vi "Move SBlock Down.vi"(8 "error in (no error)":errorcluster, 10 "index":i32, 11 "Sequence of SBlocks in":refnum<class "Sequence of SBlocks.lvclass">) -> (0 "error out":errorcluster, 2 "New Index":i32, 3 "Sequence of SBlocks out":refnum<class "Sequence of SBlocks.lvclass">)   [LabVIEW 2020, in "Run Utilities.lvlib" / "Sequence of SBlocks.lvclass"]
uses:
  Sequence of SBlocks.lvclass
  Sequence of SBlocks.lvclass/Sequence of SBlocks.ctl
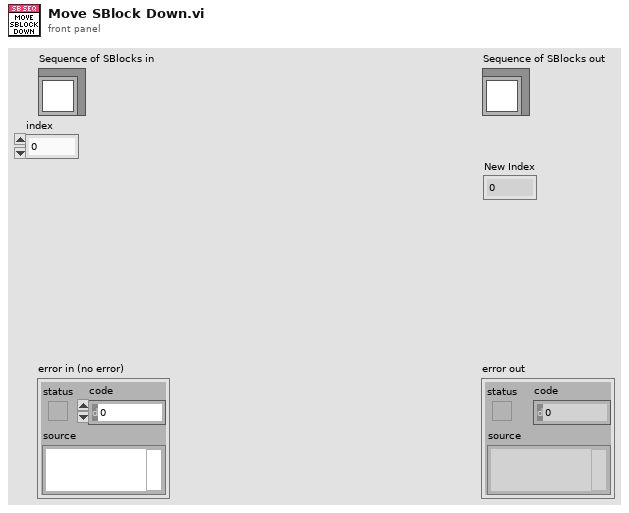
[diagram p1: front panel]
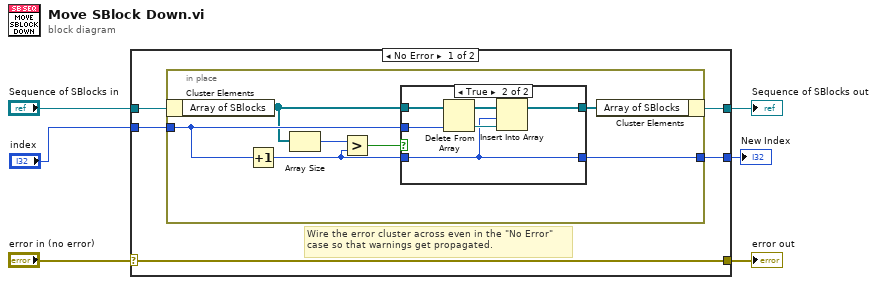
[diagram p0: block diagram]
diagram:
  n1 = case shown="No Error" "error in (no error)" {
    selector: "error in (no error)" -> [w11 w29]
    tunnel: [w11 w29] -> w5
    tunnel: [w9 w28] -> w3
    tunnel: "Sequence of SBlocks in" -> [w10 w28]
    tunnel: "index" -> [w8 w27]
    tunnel: [w7 w27] -> w1
    frame No Error {
      # "Wire the error cluster across even in the \"No Error\"\ncase so that warnings get propagated."
      n2 = in-place {
        in-place-border: w8 -> [w18]
        in-place-border: [w16] -> w7
        n3 = in-place-cluster #1(w10) -> ("Array of SBlocks"=w15:refnum<class "Schedule Block.lvclass">[])
        n4 = Increment(x=w18) -> (x+1=w13:i32)
        n5 = Array Size(array=w15) -> (size(s)=w14:i32)
        n6 = Greater?(x=w14, y=w13) -> (0:w12:bool)
        n7 = case shown="True" w12 {
          tunnel: w15 -> [w20 w26]
          tunnel: w18 -> [w19 w23]
          tunnel: [w20 w22] -> w17
          tunnel: w13 -> [_ w21]
          tunnel: [w19 w21] -> w16
          frame False {
          }
          frame True {
            n8 = Delete From Array(array=w26, index=w23) -> (deleted portion=w24:refnum<class "Schedule Block.lvclass">, array with subset deleted=w25:refnum<class "Schedule Block.lvclass">[])  [unwired: 1 in]
            n9 = Insert Into Array(array=w25, index=w21, new element=w24) -> (w22:refnum<class "Schedule Block.lvclass">[])
          }
        }
        n10 = in-place-cluster #1("Array of SBlocks"=w17) -> (w9:refnum<class "Sequence of SBlocks.lvclass">)
      }
    }
    frame Error {
    }
  }
  "error out" <- w5
  "Sequence of SBlocks out" <- w3
  "New Index" <- w1
